vi "FormatDictionaryValue.vi"(1 "key":string, 2 "dictionary":string) -> (0 "python object":string)   [LabVIEW 2014, in "Python Functions.lvlib"]
uses:
  Python Functions.lvlib
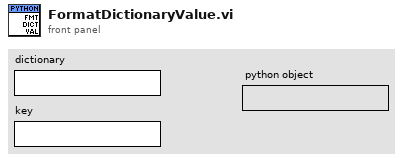
[diagram p1: front panel]
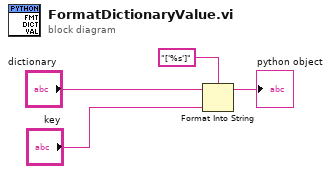
[diagram p0: block diagram]
diagram:
  n1 = Format Into String(format string="['%s']", initial string="dictionary", "key") -> (resulting string=→"python object":string)  [unwired: 1 in, 1 out]
